vi "Write value.vi"(8 "error in (no error)":errorcluster, 10 "value":string, 11 "JSON String in":refnum<class "JSON String.lvclass">) -> (0 "error out":errorcluster, 3 "JSON String out":refnum<class "JSON String.lvclass">)   [LabVIEW 2017, in "LVJSON.lvlib" / "JSON String.lvclass"]
uses:
  JSON String.lvclass
  JSON String.lvclass/JSON String.ctl
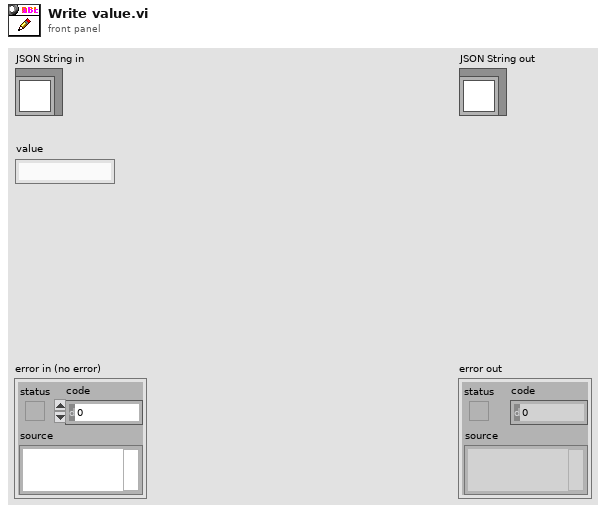
[diagram p1: front panel]
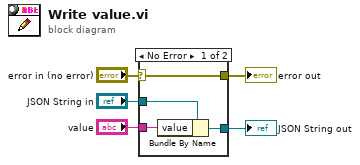
[diagram p0: block diagram]
diagram:
  n1 = case shown="No Error" "error in (no error)" {
    selector: "error in (no error)" -> [w9 w10]
    tunnel: [w9 w10] -> w4
    tunnel: [w7 w11] -> w2
    tunnel: "JSON String in" -> [w8 w11]
    tunnel: "value" -> [w6 _]
    frame No Error {
      n2 = Bundle By Name(cluster=w8, "value"=w6) -> (w7:refnum<class "JSON String.lvclass">)
    }
    frame Error {
    }
  }
  "error out" <- w4
  "JSON String out" <- w2
